vi "resetAllChannels.vi"(8 "error in (no error)":errorcluster, 11 "AtomChipHWC in":refnum<class "AtomChipHWC.lvclass">) -> (0 "error out":errorcluster, 3 "AtomChipHWC out":refnum<class "AtomChipHWC.lvclass">)   [LabVIEW 2009, in "Hardware.lvlib" / "HWControllers.lvlib" / "AtomChipHWC.lvclass"]
uses:
  AtomChipHWC.lvclass
  AtomChipHWC.lvclass/AtomChipHWC.ctl
  Channels/VoltOutput/AnalogOutput.lvclass
  Channels/Digital/DigitalOutput.lvclass
  Channels/DDSOutput/Generic/DDSOutput.lvclass
  HWController.lvclass
  Tools/DatabaseHelpers/DbConnection/DeviceDataBase/deviceDataBase.lvclass
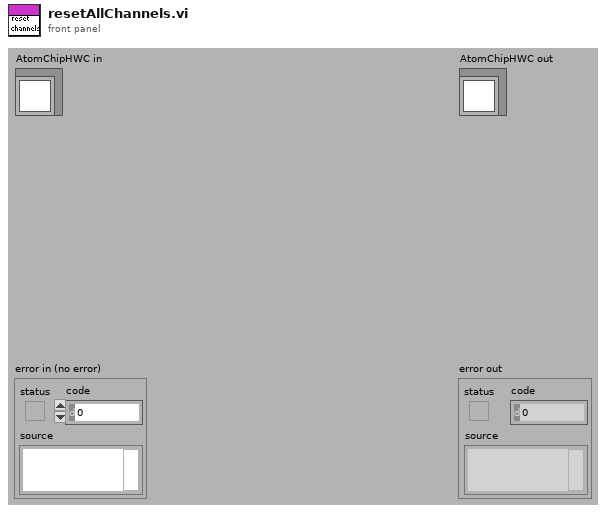
[diagram p1: front panel]
types:
  T1 = cluster{"Frequency(MHz)":dbl, "Amplitude":dbl, "Phase":dbl, "OutputForm":enum16{"Sine", "Square", "Triangle", "Arbitrary"}}[]
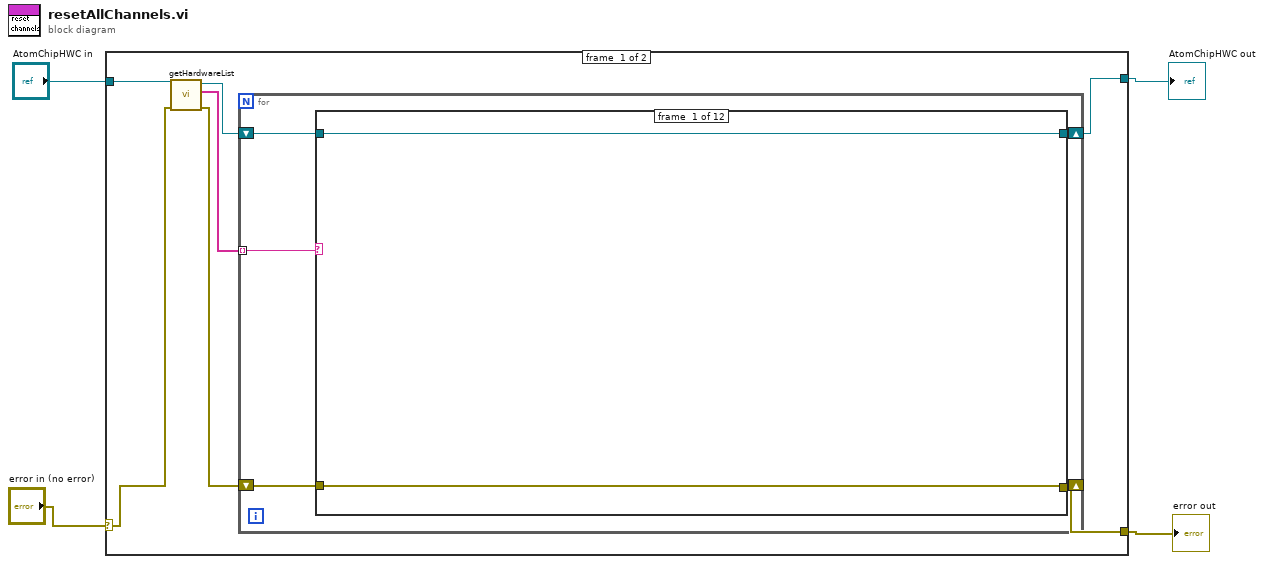
[diagram p0: block diagram]
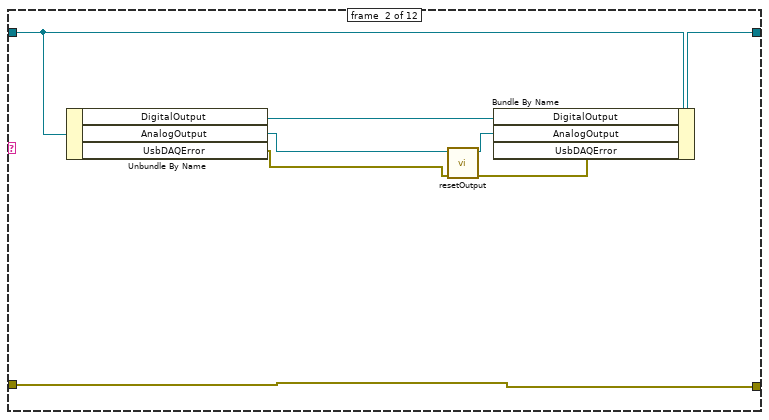
[diagram p2: hidden frame]
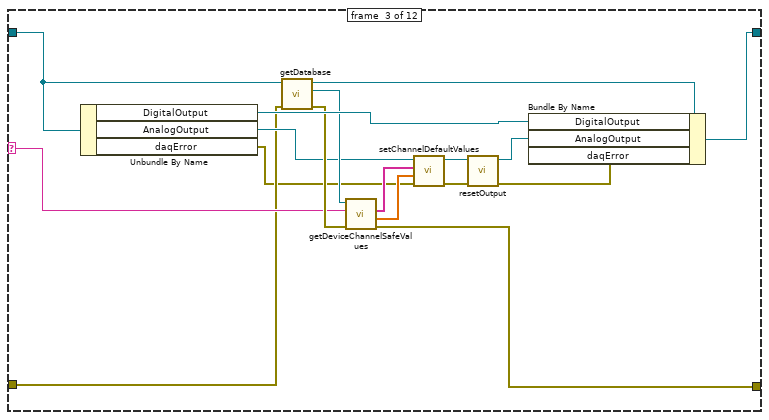
[diagram p3: hidden frame]
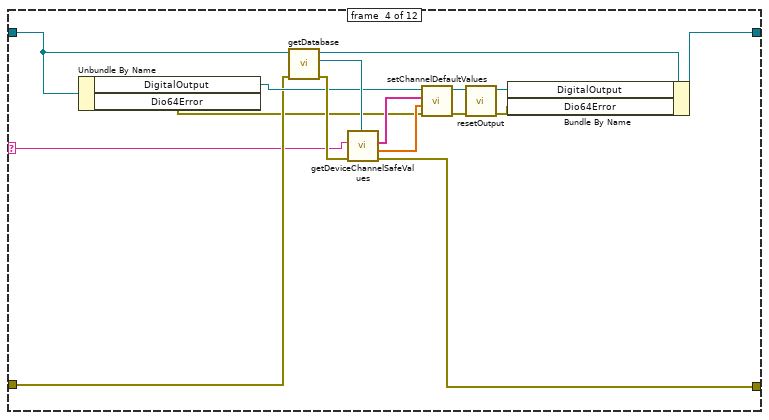
[diagram p4: hidden frame]
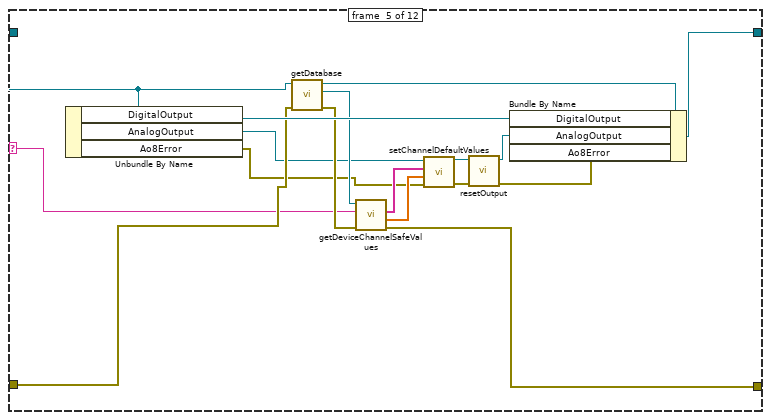
[diagram p5: hidden frame]
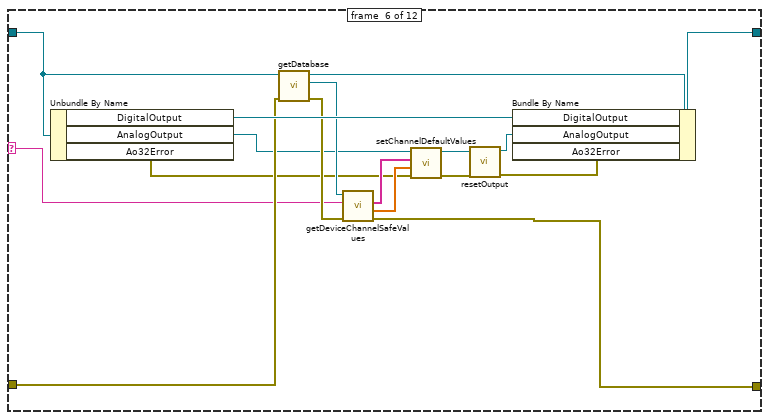
[diagram p6: hidden frame]
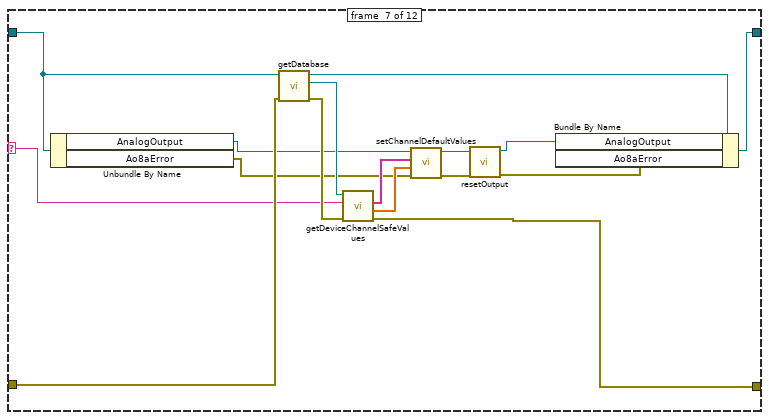
[diagram p7: hidden frame]
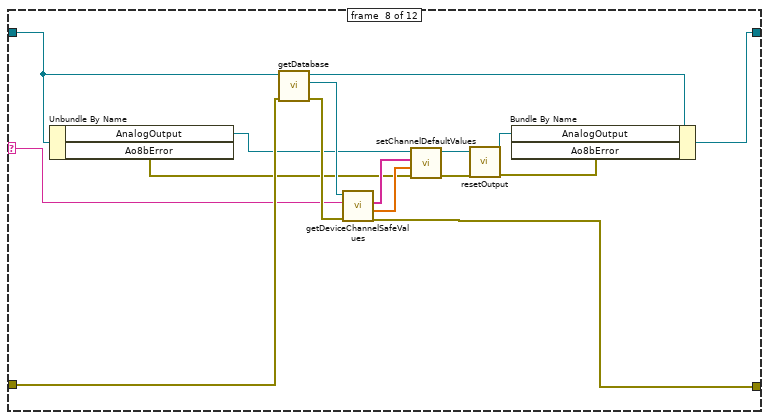
[diagram p8: hidden frame]
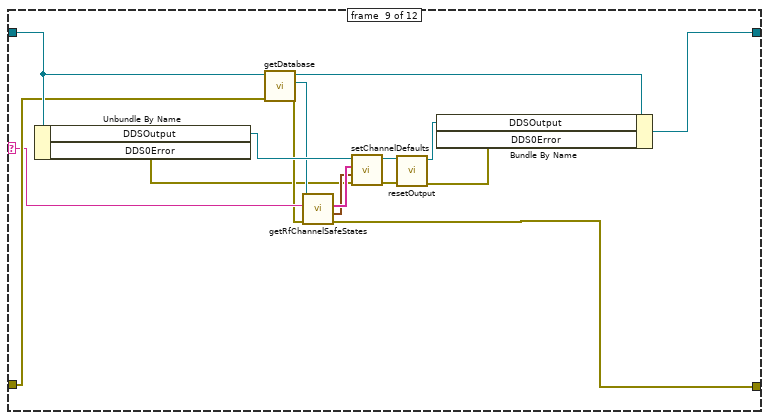
[diagram p9: hidden frame]
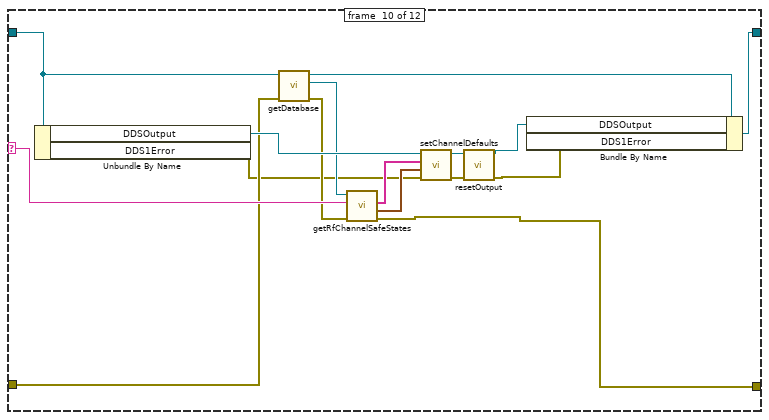
[diagram p10: hidden frame]
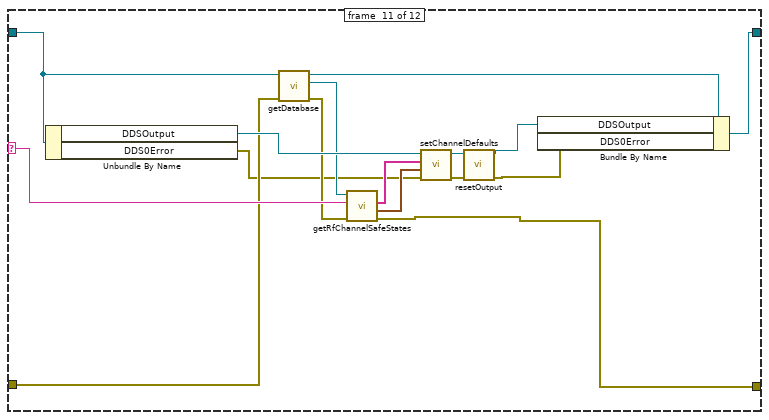
[diagram p11: hidden frame]
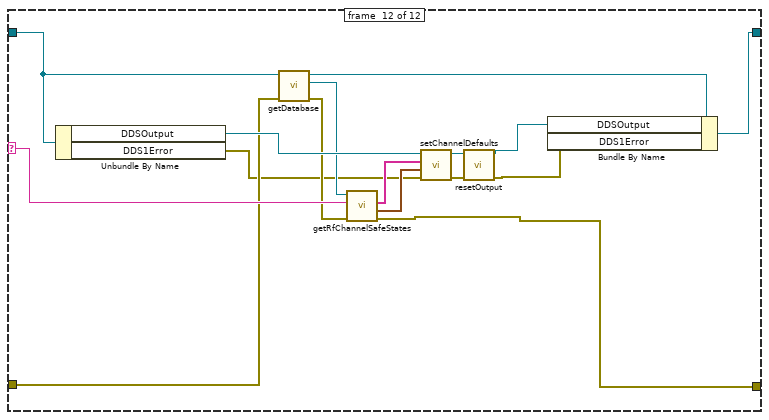
[diagram p12: hidden frame]
diagram:
  n1 = case shown="No Error" "error in (no error)" {
    selector: "error in (no error)" -> [w6 w190]
    tunnel: [w10 w190] -> w1
    tunnel: [w11 w191] -> w2
    tunnel: "AtomChipHWC in" -> [w9 w191]
    frame #0 {
      n2 = call "getHardwareList.vi"("error in (no error)"=w6, "HWController.lvclass in"=w9) -> ("error out"=w5:errorcluster, "HardwareList"=w8:string[], "HWController.lvclass out"=w7:refnum<class "AtomChipHWC.lvclass">)  [unwired: 7 in]
      n3 = for {
        tunnel: w8 -> [w13] mode=indexing
        shift-right: [w16] -> w11
        shift-left: w7 -> [w12]
        shift-right: [w14] -> w10
        shift-left: w5 -> [w15]
        n4 = case shown="\"k3390\"" w13 {
          selector: w13 -> [_ _ w32 w49 w65 w80 w97 w113 w132 w149 w165 w181]
          tunnel: w12 -> [w18 w26 w34 w53 w69 w86 w103 w119 w140 w156 w172 w188]
          tunnel: [w18 w25 w43 w59 w76 w93 w109 w125 w141 w157 w173 w189] -> w16
          tunnel: w15 -> [w17 w19 w30 w50 w67 w85 w102 w118 w139 w145 w161 w177]
          tunnel: [w17 w19 w29 w44 w60 w78 w95 w111 w127 w143 w159 w175] -> w14
          frame #0 {
          }
          frame #1 {
            n5 = Unbundle By Name(w26) -> ("DigitalOutput"=w22:refnum<class "DigitalOutput.lvclass">, "AnalogOutput"=w24:refnum<class "AnalogOutput.lvclass">, "UsbDAQError"=w21:errorcluster)
            n6 = call-dynamic "resetOutput.vi"("error in (no error)"=w21, "AnalogOutput in"=w24) -> ("error out"=w20:errorcluster, "AnalogOutput out"=w23:refnum<class "AnalogOutput.lvclass">)  [unwired: 8 in]
            n7 = Bundle By Name(cluster=w26, "DigitalOutput"=w22, "AnalogOutput"=w23, "UsbDAQError"=w20) -> (w25:refnum<class "AtomChipHWC.lvclass">)
          }
          frame #2 {
            n8 = Unbundle By Name(w34) -> ("DigitalOutput"=w41:refnum<class "DigitalOutput.lvclass">, "AnalogOutput"=w35:refnum<class "AnalogOutput.lvclass">, "daqError"=w27:errorcluster)
            n9 = call "getDatabase.vi"("error in (no error)"=w30, "HWController in"=w34) -> ("error out"=w39:errorcluster, "deviceDataBase"=w40:refnum<class "deviceDataBase.lvclass">, "HWController out"=w33:refnum<class "AtomChipHWC.lvclass">)  [unwired: 7 in]
            n10 = call "getDeviceChannelSafeValues.vi"("error in (no error)"=w39, "device_name"=w32, "deviceDataBase in"=w40) -> ("error out"=w29:errorcluster, "SafeVaues"=w38:dbl[], "ChannelAddresses"=w37:string[])  [unwired: 5 in, 1 out]
            n11 = call "setChannelDefaultValues.vi"("error in (no error)"=w27, "calibratedValues"=w38, "channel_addresses"=w37, "AnalogOutput in"=w35) -> ("error out"=w31:errorcluster, "AnalogOutput out"=w36:refnum<class "AnalogOutput.lvclass">)  [unwired: 6 in]
            n12 = call-dynamic "resetOutput.vi"("error in (no error)"=w31, "AnalogOutput in"=w36) -> ("error out"=w28:errorcluster, "AnalogOutput out"=w42:refnum<class "AnalogOutput.lvclass">)  [unwired: 8 in]
            n13 = Bundle By Name(cluster=w33, "DigitalOutput"=w41, "AnalogOutput"=w42, "daqError"=w28) -> (w43:refnum<class "AtomChipHWC.lvclass">)
          }
          frame #3 {
            n14 = Unbundle By Name(w53) -> ("DigitalOutput"=w51:refnum<class "DigitalOutput.lvclass">, "Dio64Error"=w46:errorcluster)
            n15 = call "getDatabase.vi"("error in (no error)"=w50, "HWController in"=w53) -> ("error out"=w56:errorcluster, "deviceDataBase"=w57:refnum<class "deviceDataBase.lvclass">, "HWController out"=w52:refnum<class "AtomChipHWC.lvclass">)  [unwired: 7 in]
            n16 = call "getDeviceChannelSafeValues.vi"("error in (no error)"=w56, "device_name"=w49, "deviceDataBase in"=w57) -> ("error out"=w44:errorcluster, "SafeVaues"=w54:dbl[], "ChannelAddresses"=w55:string[])  [unwired: 5 in, 1 out]
            n17 = call-dynamic "setChannelDefaultValues.vi"("error in (no error)"=w46, "calibratedValues"=w54, "channel_addresses"=w55, "DigitalOutput in"=w51) -> ("error out"=w48:errorcluster, "DigitalOutput out"=w47:refnum<class "DigitalOutput.lvclass">)  [unwired: 6 in]
            n18 = call-dynamic "resetOutput.vi"("error in (no error)"=w48, "DigitalOutput in"=w47) -> ("error out"=w45:errorcluster, "DigitalOutput out"=w58:refnum<class "DigitalOutput.lvclass">)  [unwired: 8 in]
            n19 = Bundle By Name(cluster=w52, "DigitalOutput"=w58, "Dio64Error"=w45) -> (w59:refnum<class "AtomChipHWC.lvclass">)
          }
          frame #4 {
            n20 = Unbundle By Name(w69) -> ("DigitalOutput"=w74:refnum<class "DigitalOutput.lvclass">, "AnalogOutput"=w66:refnum<class "AnalogOutput.lvclass">, "Ao8Error"=w61:errorcluster)
            n21 = call "getDatabase.vi"("error in (no error)"=w67, "HWController in"=w69) -> ("error out"=w72:errorcluster, "deviceDataBase"=w73:refnum<class "deviceDataBase.lvclass">, "HWController out"=w68:refnum<class "AtomChipHWC.lvclass">)  [unwired: 7 in]
            n22 = call "getDeviceChannelSafeValues.vi"("error in (no error)"=w72, "device_name"=w65, "deviceDataBase in"=w73) -> ("error out"=w60:errorcluster, "SafeVaues"=w71:dbl[], "ChannelAddresses"=w70:string[])  [unwired: 5 in, 1 out]
            n23 = call "setChannelDefaultValues.vi"("error in (no error)"=w61, "calibratedValues"=w71, "channel_addresses"=w70, "AnalogOutput in"=w66) -> ("error out"=w63:errorcluster, "AnalogOutput out"=w64:refnum<class "AnalogOutput.lvclass">)  [unwired: 6 in]
            n24 = call-dynamic "resetOutput.vi"("error in (no error)"=w63, "AnalogOutput in"=w64) -> ("error out"=w62:errorcluster, "AnalogOutput out"=w75:refnum<class "AnalogOutput.lvclass">)  [unwired: 8 in]
            n25 = Bundle By Name(cluster=w68, "DigitalOutput"=w74, "AnalogOutput"=w75, "Ao8Error"=w62) -> (w76:refnum<class "AtomChipHWC.lvclass">)
          }
          frame #5 {
            n26 = Unbundle By Name(w86) -> ("DigitalOutput"=w91:refnum<class "DigitalOutput.lvclass">, "AnalogOutput"=w83:refnum<class "AnalogOutput.lvclass">, "Ao32Error"=w79:errorcluster)
            n27 = call "getDatabase.vi"("error in (no error)"=w85, "HWController in"=w86) -> ("error out"=w89:errorcluster, "deviceDataBase"=w90:refnum<class "deviceDataBase.lvclass">, "HWController out"=w82:refnum<class "AtomChipHWC.lvclass">)  [unwired: 7 in]
            n28 = call "getDeviceChannelSafeValues.vi"("error in (no error)"=w89, "device_name"=w80, "deviceDataBase in"=w90) -> ("error out"=w78:errorcluster, "SafeVaues"=w88:dbl[], "ChannelAddresses"=w87:string[])  [unwired: 5 in, 1 out]
            n29 = call "setChannelDefaultValues.vi"("error in (no error)"=w79, "calibratedValues"=w88, "channel_addresses"=w87, "AnalogOutput in"=w83) -> ("error out"=w84:errorcluster, "AnalogOutput out"=w81:refnum<class "AnalogOutput.lvclass">)  [unwired: 6 in]
            n30 = call-dynamic "resetOutput.vi"("error in (no error)"=w84, "AnalogOutput in"=w81) -> ("error out"=w77:errorcluster, "AnalogOutput out"=w92:refnum<class "AnalogOutput.lvclass">)  [unwired: 8 in]
            n31 = Bundle By Name(cluster=w82, "DigitalOutput"=w91, "AnalogOutput"=w92, "Ao32Error"=w77) -> (w93:refnum<class "AtomChipHWC.lvclass">)
          }
          frame #6 {
            n32 = Unbundle By Name(w103) -> ("AnalogOutput"=w100:refnum<class "AnalogOutput.lvclass">, "Ao8aError"=w96:errorcluster)
            n33 = call "getDatabase.vi"("error in (no error)"=w102, "HWController in"=w103) -> ("error out"=w106:errorcluster, "deviceDataBase"=w107:refnum<class "deviceDataBase.lvclass">, "HWController out"=w99:refnum<class "AtomChipHWC.lvclass">)  [unwired: 7 in]
            n34 = call "getDeviceChannelSafeValues.vi"("error in (no error)"=w106, "device_name"=w97, "deviceDataBase in"=w107) -> ("error out"=w95:errorcluster, "SafeVaues"=w105:dbl[], "ChannelAddresses"=w104:string[])  [unwired: 5 in, 1 out]
            n35 = call "setChannelDefaultValues.vi"("error in (no error)"=w96, "calibratedValues"=w105, "channel_addresses"=w104, "AnalogOutput in"=w100) -> ("error out"=w101:errorcluster, "AnalogOutput out"=w98:refnum<class "AnalogOutput.lvclass">)  [unwired: 6 in]
            n36 = call-dynamic "resetOutput.vi"("error in (no error)"=w101, "AnalogOutput in"=w98) -> ("error out"=w94:errorcluster, "AnalogOutput out"=w108:refnum<class "AnalogOutput.lvclass">)  [unwired: 8 in]
            n37 = Bundle By Name(cluster=w99, "AnalogOutput"=w108, "Ao8aError"=w94) -> (w109:refnum<class "AtomChipHWC.lvclass">)
          }
          frame #7 {
            n38 = Unbundle By Name(w119) -> ("AnalogOutput"=w116:refnum<class "AnalogOutput.lvclass">, "Ao8bError"=w112:errorcluster)
            n39 = call "getDatabase.vi"("error in (no error)"=w118, "HWController in"=w119) -> ("error out"=w122:errorcluster, "deviceDataBase"=w123:refnum<class "deviceDataBase.lvclass">, "HWController out"=w115:refnum<class "AtomChipHWC.lvclass">)  [unwired: 7 in]
            n40 = call "getDeviceChannelSafeValues.vi"("error in (no error)"=w122, "device_name"=w113, "deviceDataBase in"=w123) -> ("error out"=w111:errorcluster, "SafeVaues"=w121:dbl[], "ChannelAddresses"=w120:string[])  [unwired: 5 in, 1 out]
            n41 = call "setChannelDefaultValues.vi"("error in (no error)"=w112, "calibratedValues"=w121, "channel_addresses"=w120, "AnalogOutput in"=w116) -> ("error out"=w117:errorcluster, "AnalogOutput out"=w114:refnum<class "AnalogOutput.lvclass">)  [unwired: 6 in]
            n42 = call-dynamic "resetOutput.vi"("error in (no error)"=w117, "AnalogOutput in"=w114) -> ("error out"=w110:errorcluster, "AnalogOutput out"=w124:refnum<class "AnalogOutput.lvclass">)  [unwired: 8 in]
            n43 = Bundle By Name(cluster=w115, "AnalogOutput"=w124, "Ao8bError"=w110) -> (w125:refnum<class "AtomChipHWC.lvclass">)
          }
          frame #8 {
            n44 = Unbundle By Name(w140) -> ("DDSOutput"=w137:refnum<class "DDSOutput.lvclass">, "DDS0Error"=w128:errorcluster)
            n45 = call "getDatabase.vi"("error in (no error)"=w139, "HWController in"=w140) -> ("error out"=w131:errorcluster, "deviceDataBase"=w133:refnum<class "deviceDataBase.lvclass">, "HWController out"=w138:refnum<class "AtomChipHWC.lvclass">)  [unwired: 7 in]
            n46 = call "getRfChannelSafeStates.vi"("error in (no error)"=w131, "deviceName"=w132, "deviceDataBase in"=w133) -> ("error out"=w127:errorcluster, "safestates"=w129:T1, "ChannelAddresses"=w130:string[])  [unwired: 5 in, 1 out]
            n47 = call-dynamic "setChannelDefaults.vi"("error in (no error)"=w128, "Data"=w129, "physicalChannels"=w130, "DDSOutput in"=w137) -> ("error out"=w135:errorcluster, "DDSOutput out"=w136:refnum<class "DDSOutput.lvclass">)  [unwired: 6 in]
            n48 = call-dynamic "resetOutput.vi"("error in (no error)"=w135, "DDSOutput in"=w136) -> ("error out"=w126:errorcluster, "DDSOutput out"=w134:refnum<class "DDSOutput.lvclass">)  [unwired: 8 in]
            n49 = Bundle By Name(cluster=w138, "DDSOutput"=w134, "DDS0Error"=w126) -> (w141:refnum<class "AtomChipHWC.lvclass">)
          }
          frame #9 {
            n50 = Unbundle By Name(w156) -> ("DDSOutput"=w154:refnum<class "DDSOutput.lvclass">, "DDS1Error"=w142:errorcluster)
            n51 = call "getDatabase.vi"("error in (no error)"=w145, "HWController in"=w156) -> ("error out"=w148:errorcluster, "deviceDataBase"=w150:refnum<class "deviceDataBase.lvclass">, "HWController out"=w155:refnum<class "AtomChipHWC.lvclass">)  [unwired: 7 in]
            n52 = call "getRfChannelSafeStates.vi"("error in (no error)"=w148, "deviceName"=w149, "deviceDataBase in"=w150) -> ("error out"=w143:errorcluster, "safestates"=w147:T1, "ChannelAddresses"=w146:string[])  [unwired: 5 in, 1 out]
            n53 = call-dynamic "setChannelDefaults.vi"("error in (no error)"=w142, "Data"=w147, "physicalChannels"=w146, "DDSOutput in"=w154) -> ("error out"=w152:errorcluster, "DDSOutput out"=w153:refnum<class "DDSOutput.lvclass">)  [unwired: 6 in]
            n54 = call-dynamic "resetOutput.vi"("error in (no error)"=w152, "DDSOutput in"=w153) -> ("error out"=w144:errorcluster, "DDSOutput out"=w151:refnum<class "DDSOutput.lvclass">)  [unwired: 8 in]
            n55 = Bundle By Name(cluster=w155, "DDSOutput"=w151, "DDS1Error"=w144) -> (w157:refnum<class "AtomChipHWC.lvclass">)
          }
          frame #10 {
            n56 = Unbundle By Name(w172) -> ("DDSOutput"=w170:refnum<class "DDSOutput.lvclass">, "DDS0Error"=w158:errorcluster)
            n57 = call "getDatabase.vi"("error in (no error)"=w161, "HWController in"=w172) -> ("error out"=w164:errorcluster, "deviceDataBase"=w166:refnum<class "deviceDataBase.lvclass">, "HWController out"=w171:refnum<class "AtomChipHWC.lvclass">)  [unwired: 7 in]
            n58 = call "getRfChannelSafeStates.vi"("error in (no error)"=w164, "deviceName"=w165, "deviceDataBase in"=w166) -> ("error out"=w159:errorcluster, "safestates"=w163:T1, "ChannelAddresses"=w162:string[])  [unwired: 5 in, 1 out]
            n59 = call-dynamic "setChannelDefaults.vi"("error in (no error)"=w158, "Data"=w163, "physicalChannels"=w162, "DDSOutput in"=w170) -> ("error out"=w168:errorcluster, "DDSOutput out"=w169:refnum<class "DDSOutput.lvclass">)  [unwired: 6 in]
            n60 = call-dynamic "resetOutput.vi"("error in (no error)"=w168, "DDSOutput in"=w169) -> ("error out"=w160:errorcluster, "DDSOutput out"=w167:refnum<class "DDSOutput.lvclass">)  [unwired: 8 in]
            n61 = Bundle By Name(cluster=w171, "DDSOutput"=w167, "DDS0Error"=w160) -> (w173:refnum<class "AtomChipHWC.lvclass">)
          }
          frame #11 {
            n62 = Unbundle By Name(w188) -> ("DDSOutput"=w186:refnum<class "DDSOutput.lvclass">, "DDS1Error"=w174:errorcluster)
            n63 = call "getDatabase.vi"("error in (no error)"=w177, "HWController in"=w188) -> ("error out"=w180:errorcluster, "deviceDataBase"=w182:refnum<class "deviceDataBase.lvclass">, "HWController out"=w187:refnum<class "AtomChipHWC.lvclass">)  [unwired: 7 in]
            n64 = call "getRfChannelSafeStates.vi"("error in (no error)"=w180, "deviceName"=w181, "deviceDataBase in"=w182) -> ("error out"=w175:errorcluster, "safestates"=w179:T1, "ChannelAddresses"=w178:string[])  [unwired: 5 in, 1 out]
            n65 = call-dynamic "setChannelDefaults.vi"("error in (no error)"=w174, "Data"=w179, "physicalChannels"=w178, "DDSOutput in"=w186) -> ("error out"=w184:errorcluster, "DDSOutput out"=w185:refnum<class "DDSOutput.lvclass">)  [unwired: 6 in]
            n66 = call-dynamic "resetOutput.vi"("error in (no error)"=w184, "DDSOutput in"=w185) -> ("error out"=w176:errorcluster, "DDSOutput out"=w183:refnum<class "DDSOutput.lvclass">)  [unwired: 8 in]
            n67 = Bundle By Name(cluster=w187, "DDSOutput"=w183, "DDS1Error"=w176) -> (w189:refnum<class "AtomChipHWC.lvclass">)
          }
        }
      }
    }
    frame #1 {
    }
  }
  "error out" <- w1
  "AtomChipHWC out" <- w2
